vi "Vibration Analysis (SubVI).vi"(8 "data":waveform(dbl), 9 "RMS Threshold":dbl, 10 "Max-Min Threshold":dbl, 11 "Cluster":T1) -> (3 "output cluster":T1={"Vibration Wfm Data"={"t0"=timestamp(3614627182.308542 s since 1904-01-01), "dt"=0.0, "Y"=array[51200 elements], "attributes"=variant("NI_ChannelName"=variant(string "Mod1/ai0"), "NI_UnitDescription"=variant(string "Volts"))}, "RMS"=0.0, "Max-Min"=0.0, "RMS Alarm"=FALSE, "Max-Min Alarm"=FALSE, "Vibration Alarm"=FALSE, "Chamber Name"=""})   [LabVIEW 2017]
uses:
  Vibration.ctl
  <vilib>/addons/_NISVFA/_Shared subVIs/Controls/svc_Engineering Units Text Ring.ctl
  <vilib>/addons/_NISVFA/_Shared subVIs/Controls/svc_Weighting Filter Text Ring.ctl
  <vilib>/addons/Sound and Vibration/svt_Calibration/SVL Scale Voltage to EU (1 Ch).vi
  <vilib>/addons/_NISVFA/_Shared subVIs/Common/svc_Set SV Channel Info.vi
  <vilib>/addons/_NISVFA/_Shared subVIs/Common/svc_Set SV Channel Info (variant).vi
  <vilib>/addons/_NISVFA/_Shared subVIs/Common/SVL Set dB Reference (variant).vi
  <vilib>/addons/_NISVFA/_Shared subVIs/Common/svc_Engineering Units to Unit Label.vi
  <vilib>/addons/_NISVFA/_Shared subVIs/Common/svc_Compute Scale Factor to Convert V to EU.vi
  <vilib>/addons/_NISVFA/_Shared subVIs/Common/svc_Compute Scale Factor to Convert C to EU.vi
  <vilib>/addons/_NISVFA/_Shared subVIs/Common/svc_Set dB ref if Pascal.vi
  <vilib>/addons/_NISVFA/_Shared subVIs/Common/svc_Caller VI Returned in Error Source.vi
  <vilib>/addons/Sound and Vibration/svt_Level/SVL Max-Min Level (1 Ch).vi
  <vilib>/addons/Sound and Vibration/svt_Level/SVL Running RMS Level (1 Ch).vi
  <vilib>/addons/Sound and Vibration/svt_Calibration/SoundVib_Calibration.lvlib
  <vilib>/addons/Sound and Vibration/svt_Level/SoundVib_VibrationLevel.lvlib
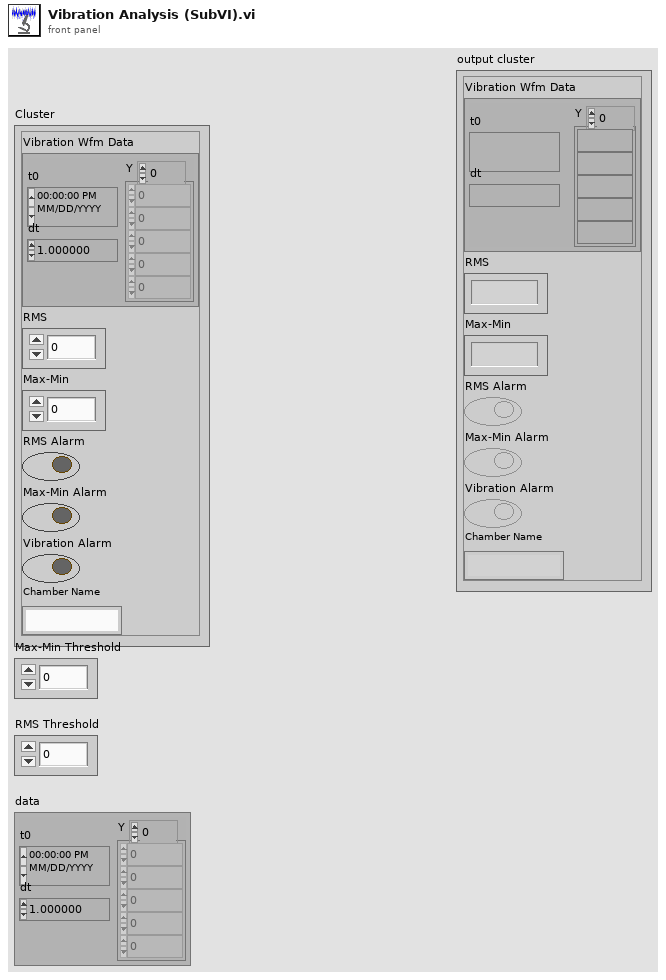
[diagram p1: front panel]
types:
  T1 = typedef "Vibration.ctl" = cluster{"Vibration Wfm Data":waveform(dbl), "RMS":dbl, "Max-Min":dbl, "RMS Alarm":bool, "Max-Min Alarm":bool, "Vibration Alarm":bool, "Chamber Name":string}
  T2 = typedef "svc_Engineering Units Text Ring.ctl" = u16
  T3 = typedef "svc_Weighting Filter Text Ring.ctl" = u16
  T4 = cluster{"sensor sensitivity":dbl, "engineering units":T2, "dB reference":dbl, "custom label":string, "weighting filter":T3, "pregain":dbl}
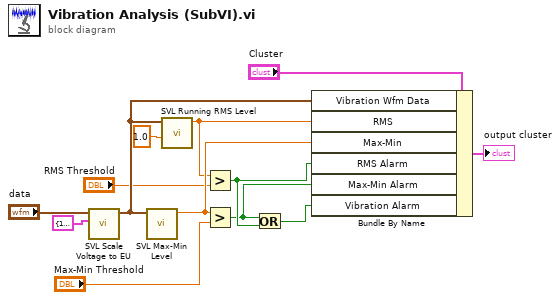
[diagram p0: block diagram]
diagram:
  n1 = call-poly <vilib>:"SVL Scale Voltage to EU.vi"("channel info"=T4 {"sensor sensitivity"=1000.0, "engineering units"=1, "dB reference"=1.0, "custom label"="EU", "weighting filter"=0, "pregain"=0.0} ("Vibration Channel Info"), "signal [V]"="data") -> ("scaled signal [EU]"=w8:waveform(dbl))  [unwired: 7 in, 2 out]
  n2 = call-poly <vilib>:"SVL Max-Min Level.vi"("scaled signal [EU]"=w8) -> ("max-min level [EU]"=w10:dbl)  [unwired: 6 in, 4 out]
  n3 = call-poly <vilib>:"SVL Running RMS Level.vi"("integration time [s]"=1.0, "scaled signal [EU]"=w8) -> ("running RMS level [EU rms]"=w9:dbl)  [unwired: 6 in, 3 out]
  n4 = Greater?(x=w9, y="RMS Threshold") -> (0:w12:bool)
  n5 = Greater?(x=w10, y="Max-Min Threshold") -> (0:w11:bool)
  n6 = Or(x=w11, y=w12) -> (x .or. y?=w13:bool)
  n7 = Bundle By Name(cluster="Cluster", "Vibration Wfm Data"=w8, "RMS"=w9, "Max-Min"=w10, "RMS Alarm"=w12, "Max-Min Alarm"=w11, "Vibration Alarm"=w13) -> (→"output cluster":T1)
